vi "Continuous Initiate.vi"(8 "error in (no error)":errorcluster, 9 "Enable Initiate Continuous (T: Enable)":bool=TRUE, 10 "Channel (1: 1)":i32(ring)=1 items=["1"=1, "2"=2, "Both"=3], 11 "VISA resource name":refnum<visa-resource-name>) -> (0 "error out":errorcluster, 3 "VISA resource name out":refnum<visa-resource-name>)   [LabVIEW 2013, in "AWG.lvlib" / "Agilent 3352X Series.lvlib"]
doc: "Initiates a continuous trigger for specified channel. \n\n<b>Note</b>:\n(1) This VI is intended to be used in pair:\nenable initiate continuous -> do something -> disable initiate continuous"
uses:
  Agilent 3352X Series.lvlib
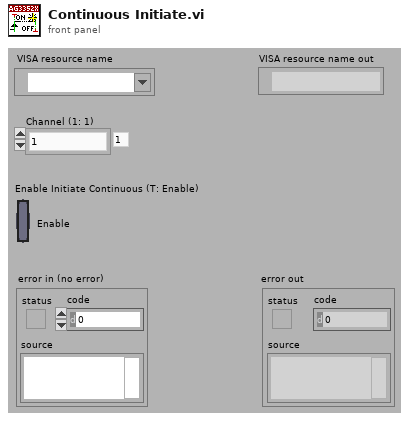
[diagram p1: front panel]
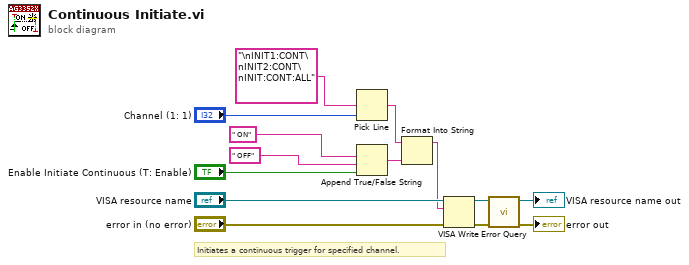
[diagram p0: block diagram]
diagram:
  # "Initiates a continuous trigger for specified channel."
  n1 = Pick Line(multi-line string="\nINIT1:CONT\nINIT2:CONT\nINIT:CONT:ALL", line index="Channel (1: 1)") -> (output string=w2:string)  [unwired: 1 out]
  n2 = Append True/False String(1:"Enable Initiate Continuous (T: Enable)", 2:" OFF", 3:" ON") -> (0:w3:string)  [unwired: 1 out]
  n3 = Format Into String(initial string=w2, w3) -> (resulting string=w1:string)  [unwired: 2 in, 1 out]
  n4 = VISA Write(VISA resource name="VISA resource name", write buffer=w1, error in (no error)="error in (no error)") -> (VISA resource name out=w7:refnum<visa-resource-name>, error out=w6:errorcluster)  [unwired: 1 out]
  n5 = call "Error Query.vi"("error in (no error)"=w6, "VISA resource name"=w7) -> ("error out"=→"error out":errorcluster, "VISA resource name out"=→"VISA resource name out":refnum<visa-resource-name>)  [unwired: 8 out]
